vi "stop.vi"(8 "error in (no error)":errorcluster, 11 "ImageAssemblerDL090211Frame in":refnum<class "ImageAssemblerDL090211Frame.lvclass">) -> (0 "error out":errorcluster, 3 "ImageAssemblerDL090211Frame out":refnum<class "ImageAssemblerDL090211Frame.lvclass">)   [LabVIEW 2010, in "ImageAssemblerDL090211Frame.lvclass"]
uses:
  ImageAssemblerDL090211Frame.lvclass
  ImageAssemblerDL090211Scaffold/ImageAssemblerDL090211Scaffold/ImageAssemblerDL090211Scaffold.lvclass
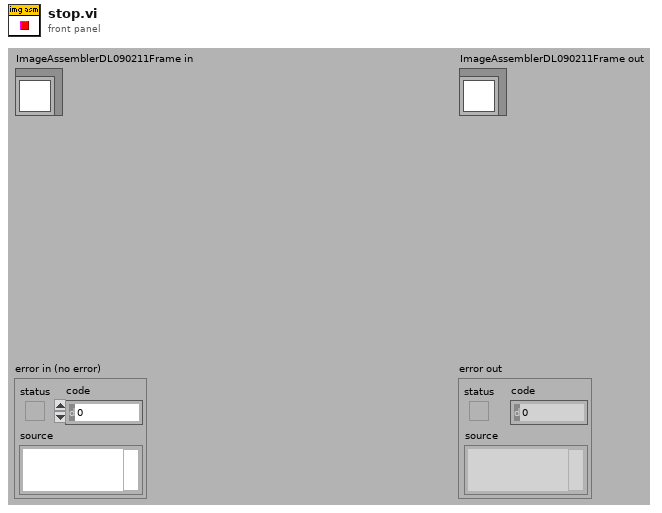
[diagram p1: front panel]
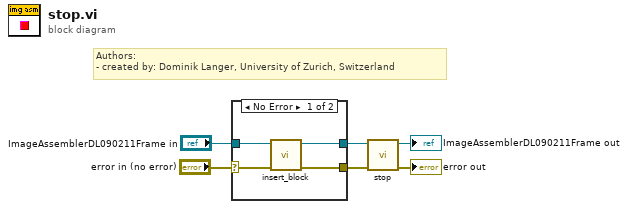
[diagram p0: block diagram]
diagram:
  # "Authors: \n- created by: Dominik Langer, University of Zurich, Switzerland"
  n1 = case shown="No Error" "error in (no error)" {
    selector: "error in (no error)" -> [w7 w11]
    tunnel: [w10 w11] -> w4
    tunnel: "ImageAssemblerDL090211Frame in" -> [w9 w12]
    tunnel: [w8 w12] -> w2
    frame No Error {
      n2 = call-dynamic "insert_block.vi"("error in (no error)"=w7, "ImageAssemblerDL090211Frame in"=w9) -> ("error out"=w10:errorcluster, "ImageAssemblerDL090211Frame out"=w8:refnum<class "ImageAssemblerDL090211Frame.lvclass">)  [unwired: 8 in]
    }
    frame Error {
    }
  }
  n3 = call-parent "stop.vi"("error in (no error)"=w4, "GenericToplevelComponent in"=w2) -> ("error out"=→"error out":errorcluster, "GenericToplevelComponent out"=→"ImageAssemblerDL090211Frame out":refnum<class "ImageAssemblerDL090211Frame.lvclass">)  [unwired: 8 in]
